vi "clase1.vi"() -> ()   [LabVIEW 2020]
panel:
  out "Numeric 3":dbl
  in  "altura":dbl
  in  "base":dbl
  out "Meter":dbl(knob) scale=0.0..100.0
  in  "Slide":dbl(slide) scale=0.0..100.0
  out "Thermometer":dbl(slide) scale=0.0..100.0
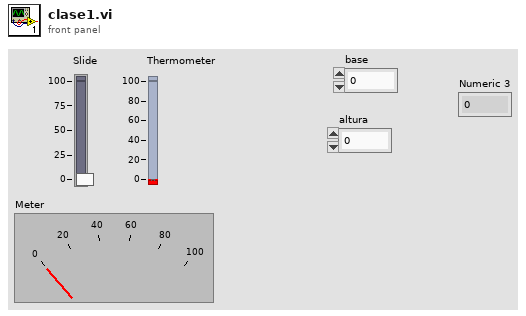
[diagram p1: front panel]
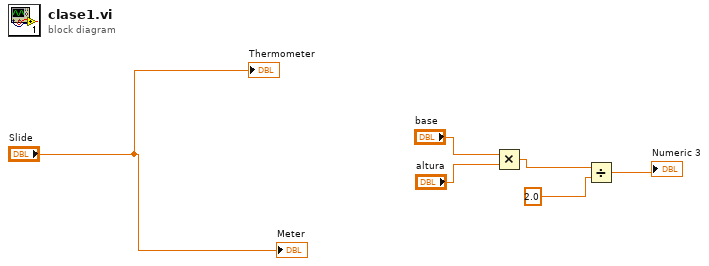
[diagram p0: block diagram]
diagram:
  n1 = Multiply(x="base", y="altura") -> (x*y=w4:dbl)
  n2 = Divide(x=w4, y=2.0) -> (x/y=→"Numeric 3":dbl)
  "Thermometer" <- "Slide"
  "Meter" <- "Slide"
